vi "test_scd_AcqStart.vi"(8 "error in":errorcluster, 11 "SCD in":refnum<class "SCD.lvclass">) -> (0 "error out":errorcluster, 3 "SCD out":refnum<class "SCD.lvclass">)   [LabVIEW 2023, in "horiba.test.lvlib"]
uses:
  horiba.test.lvlib
  Classes/SCD/SCD.lvclass
  Classes/SCD/acqSet.ctl
  1a209038-51a4-4f6a-ac39-8f9a875fcd1b.vi
  8b561903-a0cb-41fa-a950-73f271935c22.vi
  <vilib>/addons/_JKI Toolkits/Caraya/classes/Assert/Assert Equal Value_Variant.vi
  <vilib>/addons/_JKI Toolkits/Caraya/classes/Assert/Assert Less_Variant.vi
  <vilib>/addons/_JKI Toolkits/Caraya/classes/Test/Test.lvclass
  <vilib>/addons/_JKI Toolkits/Caraya/classes/Assert/Assert.lvclass
  <userlib>/_OpenG.lib/lvdata/lvdata.llb/openg_variant.lvlib
panel:
  # "Connector Pane"
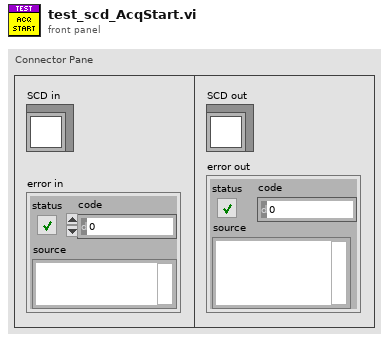
[diagram p1: front panel]
types:
  T1 = typedef "horiba.lvlib/SCD.lvclass/acqSet.ctl" = cluster{"scan_count":i32, "time_step":i32, "integration_time":i32, "external_param":i32}
  T2 = cluster{"currentSignal":cluster{"unit":string, "value":dbl}, "elapsedTime":dbl, "event_marker":bool, "overscale_current_channel":bool, "overscale_voltage_channel":bool, "pmtSignal":cluster{"unit":string, "value":dbl}, "pointNumber":dbl, "ppdSignal":cluster{"unit":string, "value":dbl}, "voltageSignal":cluster{"unit":string, "value":dbl}}[]
  T3 = cluster{"currentSignal":cluster{"unit":string, "value":dbl}, "elapsedTime":dbl, "event_marker":bool, "overscale_current_channel":bool, "overscale_voltage_channel":bool, "pmtSignal":cluster{"unit":string, "value":dbl}, "pointNumber":dbl, "ppdSignal":cluster{"unit":string, "value":dbl}, "voltageSignal":cluster{"unit":string, "value":dbl}}
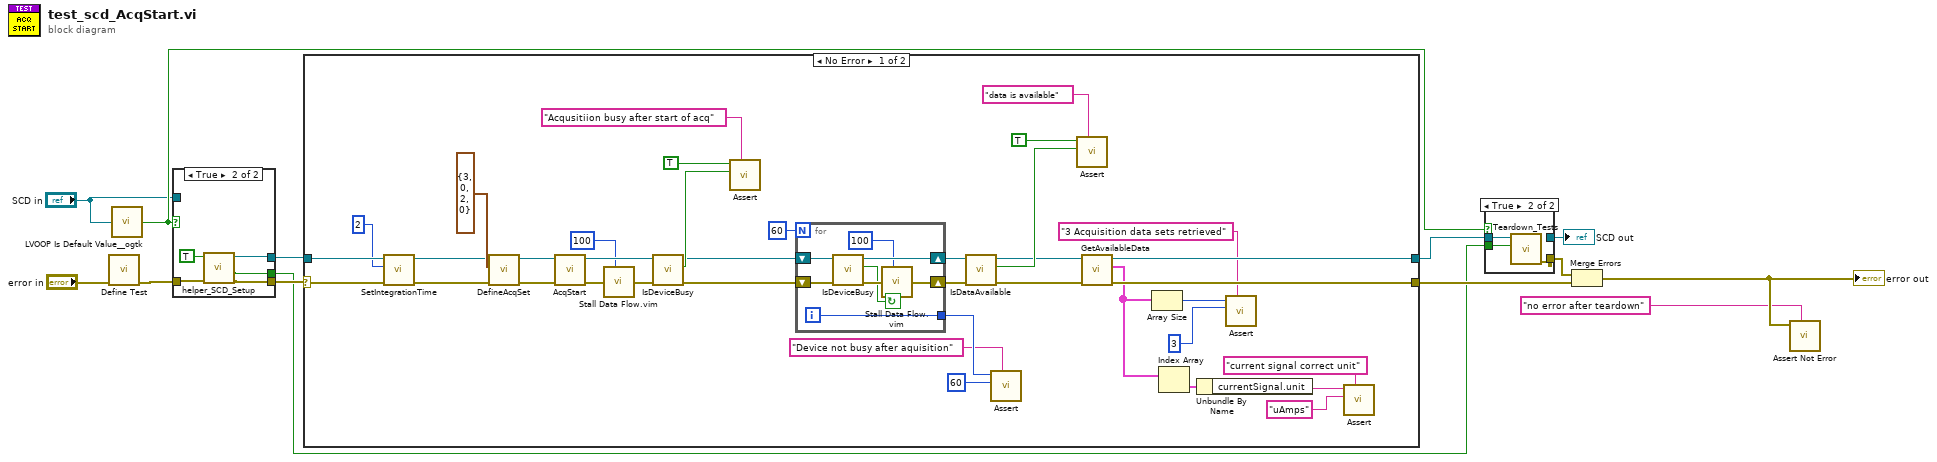
[diagram p0: block diagram]
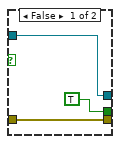
[diagram p3: hidden frame]
diagram:
  n1 = call <vilib>:"Define Test.vi"("error in (no error)"="error in") -> ("error out"=w9:errorcluster)  [unwired: 9 in, 1 out]
  n2 = call <userlib>:"LVOOP Is Default Value__ogtk.vi"("Object"="SCD in") -> ("Is Default Value?"=w3:bool)
  n3 = case shown="True" w3 {
    tunnel: w9 -> [w16 w19]
    tunnel: [w16 w21] -> w8
    tunnel: [w14 w18] -> w7
    tunnel: [TRUE ("Module Was Already Running?") w20] -> w4
    tunnel: "SCD in" -> [w14 _]
    frame False {
    }
    frame True {
      n4 = call "helper_SCD_Setup.vi"("error in"=w19, "show ICL for debugging"=TRUE) -> ("error out"=w21:errorcluster, "Module Was Already Running?"=w20:bool, "SCD out"=w18:refnum<class "SCD.lvclass">)  [unwired: 6 in, 1 out]
    }
  }
  n5 = case shown="No Error" w8 {
    selector: w8 -> [w59 w69]
    tunnel: [w41 w68] -> w12
    tunnel: w7 -> [w39 w68]
    tunnel: [w43 w69] -> w11
    frame No Error {
      n6 = call "SetIntegrationTime.vi"("error in (no error)"=w59, "integration_time"=2, "SCD in"=w39) -> ("error out"=w40:errorcluster, "SCD out"=w38:refnum<class "SCD.lvclass">)  [unwired: 7 in]
      n7 = call "DefineAcqSet.vi"("error in (no error)"=w40, "integration_time"=T1 {"scan_count"=3, "time_step"=0, "integration_time"=2, "external_param"=0}, "SCD in"=w38) -> ("error out"=w57:errorcluster, "SCD out"=w55:refnum<class "SCD.lvclass">)  [unwired: 7 in]
      n8 = call "AcqStart.vi"("error in (no error)"=w57, "SCD in"=w55) -> ("error out"=w56:errorcluster, "SCD out"=w53:refnum<class "SCD.lvclass">)  [unwired: 8 in]
      n9 = call "Stall Data Flow.vim"("value in"=w56, "milliseconds to wait"=u32 100) -> ("value out"=w52:errorcluster)  [unwired: 1 out]
      n10 = call "IsDeviceBusy.vi"("error in (no error)"=w52, "SCD in"=w53) -> ("error out"=w35:errorcluster, "isBusy"=w50:bool, "SCD out"=w47:refnum<class "SCD.lvclass">)  [unwired: 7 in]
      n11 = call-poly <vilib>:"Assert.vi"("Label"="Acqusitiion busy after start of acq", "Y"=w50, "X"=TRUE) -> ()  [unwired: 7 in, 2 out]
      n12 = for {
        N: 60 -> [_]
        shift-right: [w66] -> w36
        shift-left: w47 -> [w67]
        shift-right: [w62] -> w34
        shift-left: w35 -> [w65]
        tunnel: [w60] -> w24
        i -> [w60]
        stop <- w63 continue-if-true
        n13 = call "IsDeviceBusy.vi"("error in (no error)"=w65, "SCD in"=w67) -> ("error out"=w64:errorcluster, "isBusy"=w63:bool, "SCD out"=w66:refnum<class "SCD.lvclass">)  [unwired: 7 in]
        n14 = call "Stall Data Flow.vim"("value in"=w64, "milliseconds to wait"=u32 100) -> ("value out"=w62:errorcluster)  [unwired: 1 out]
      }
      n15 = call "IsDataAvailable.vi"("error in (no error)"=w34, "SCD in"=w36) -> ("error out"=w48:errorcluster, "isDataAvailable?"=w44:bool, "SCD out"=w42:refnum<class "SCD.lvclass">)  [unwired: 7 in]
      n16 = call-poly <vilib>:"Assert.vi"("Label"="Device not busy after aquisition", "Y"=60, "X"=w24) -> ()  [unwired: 7 in, 2 out]
      n17 = call-poly <vilib>:"Assert.vi"("Label"="data is available", "Y"=w44, "X"=TRUE) -> ()  [unwired: 7 in, 2 out]
      n18 = call "GetAvailableData.vi"("error in (no error)"=w48, "SCD in"=w42) -> ("error out"=w43:errorcluster, "data"=w29:T2, "SCD out"=w41:refnum<class "SCD.lvclass">)  [unwired: 7 in]
      n19 = Array Size(array=w29) -> (size(s)=w32:i32)
      n20 = Index Array(array=w29) -> (element=w28:T3)  [unwired: 1 in]
      n21 = Unbundle By Name(w28) -> ("currentSignal.unit"=w27:string)
      n22 = call-poly <vilib>:"Assert.vi"("Label"="3 Acquisition data sets retrieved", "Y"=3 ("size(s)"), "X"=w32) -> ()  [unwired: 7 in, 2 out]
      n23 = call-poly <vilib>:"Assert.vi"("Label"="current signal correct unit", "Y"="uAmps", "X"=w27) -> ()  [unwired: 7 in, 2 out]
    }
    frame Error {
    }
  }
  n24 = case shown="True" w3 {
    tunnel: w12 -> [w70 w73]
    tunnel: [_ w72] -> w6
    tunnel: w4 -> [_ w71]
    tunnel: [w70 _] -> w1
    frame False {
    }
    frame True {
      n25 = call "Teardown_Tests.vi"("Module Was Already Running?"=w71, "horiba.lvlib:GenericDevice"=w73) -> ("error out"=w72:errorcluster)  [unwired: 8 in, 1 out]
    }
  }
  "SCD out" <- w1
  n26 = Merge Errors(w6, w11) -> (w10:errorcluster)
  "error out" <- w10
  n27 = call <vilib>:"Assert Not Error.vi"("Label"="no error after teardown", "Not Error?"=w10) -> ()  [unwired: 8 in, 2 out]
